vi "User Events - FGV.vi"(7 "FGV States":T2, 8 "error in":errorcluster) -> (0 "error out":errorcluster, 3 "User Events Cluster":T1)   [LabVIEW 2024, in "User Events.lvlib"]
uses:
  User Events.lvlib
  General Type Defs/FGV States.ctl
  General Type Defs/User Events Cluster.ctl
  General Type Defs/General Type Defs.lvlib
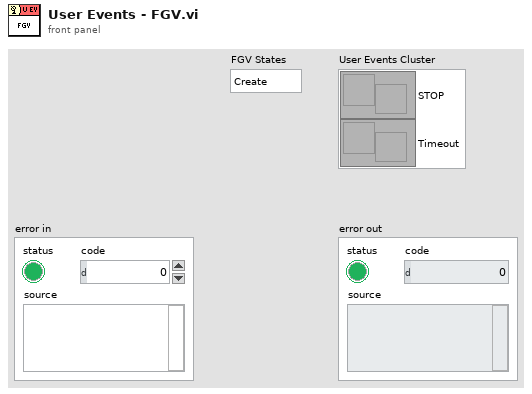
[diagram p1: front panel]
types:
  T1 = typedef "General Type Defs.lvlib/User Events Cluster.ctl" = cluster{"STOP":refnum<user-event>, "Timeout":refnum<user-event>}
  T2 = typedef "General Type Defs.lvlib/FGV States.ctl" = enum16{"Create", "Get", "Destroy"}
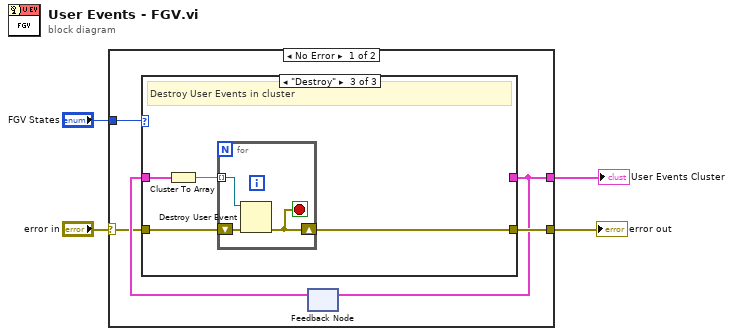
[diagram p0: block diagram]
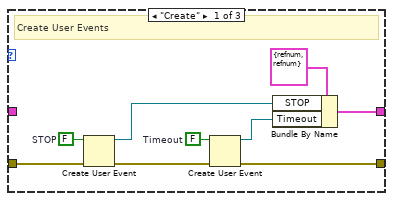
[diagram p2: hidden frame]
diagram:
  n1 = case shown="No Error" "error in" {
    selector: "error in" -> [w5 w28]
    tunnel: "FGV States" -> [w9 _]
    tunnel: [w8 w28] -> w3
    tunnel: [w6 _] -> w2
    frame No Error {
      n2 = feedback #1() -> (w7:T1)  [unwired: 1 in]
      n3 = case shown="\"Destroy\"" w9 {
        tunnel: [w12 w19 w22] -> w8
        tunnel: w5 -> [w11 w19 w21]
        tunnel: [w10 w20 _] -> w6
        tunnel: w7 -> [_ w20 w24]
        frame "Create" {
          w15 = FALSE  # Timeout
          w16 = FALSE  # STOP
          # "Create User Events"
          n4 = Create User Event(user event datatype=w16, error in=w11) -> (user event=w14:refnum<user-event>, error out=w17:errorcluster)
          n5 = Create User Event(user event datatype=w15, error in=w17) -> (user event=w13:refnum<user-event>, error out=w12:errorcluster)
          n6 = Bundle By Name(cluster=T1 {"STOP"=refnum, "Timeout"=refnum} ("User Events Cluster"), "STOP"=w14, "Timeout"=w13) -> (w10:T1)
        }
        frame "Get", Default {
          # "Get User Events"
        }
        frame "Destroy" {
          # "Destroy User Events in cluster"
          n7 = Cluster To Array(cluster=w24) -> (array=w23:refnum<user-event>[])
          n8 = for {
            tunnel: w23 -> [w27] mode=indexing
            shift-right: [w25] -> w22
            shift-left: w21 -> [w26]
            stop <- w25 stop-if-true
            n9 = Destroy User Event(user event=w27, error in=w26) -> (error out=w25:errorcluster)
          }
        }
      }
      n10 = feedback-in #1(w6) -> ()
    }
    frame Error {
    }
  }
  "User Events Cluster" <- w2
  "error out" <- w3
